vi "MenuProb.vi"(11 "Menu out":refnum<class "Menu.lvclass">) -> (2 "Value String":string, 3 "Boolean":bool)   [LabVIEW 2021, in "Menu.lvlib" / "Menu.lvclass"]
uses:
  Menu.lvclass
  Data.ctl
  Picture2D/src/Color/Color.lvclass
  Picture2D/src/Font/Font.lvclass
  Picture2D/src/Picture2D/Picture2D.lvclass
  MenuItems.ctl
  <vilib>/Utility/miscctls.llb/LVMenuShortCut.ctl
  Picture2D/src/Picture/Image.lvclass
  MenuSelection.ctl
  TD_CloseEvent.ctl
  MenuColors.ctl
  SubMenuIcon.ctl
panel:
  out "data value":T1={"MenuMap"={}, "PictRef"=refnum, "MenuSelectionEvent"=refnum, "TopMenuSpacing"=3, "MenuSpacing"=10, "CloseEvent"=refnum, "TR_ManageMenuRef"=refnum, "MenuColors"={"Text"=refnum, "HiliteText"=refnum, "Background"=refnum, "BorderColor"=refnum, "Hilite"=refnum}, "RTMPath"=path "", "RTMVIReference"=refnum, "RTMMenuReference"=refnum, "CtlRef"=refnum, "User-Specified Font"=refnum, "Desired Font"=enum."Application Font", "SubMenuIcon"=enum."LabVIEW", "SubMenuIconClosed"=refnum, "SubMenuIconOpened"=refnum}
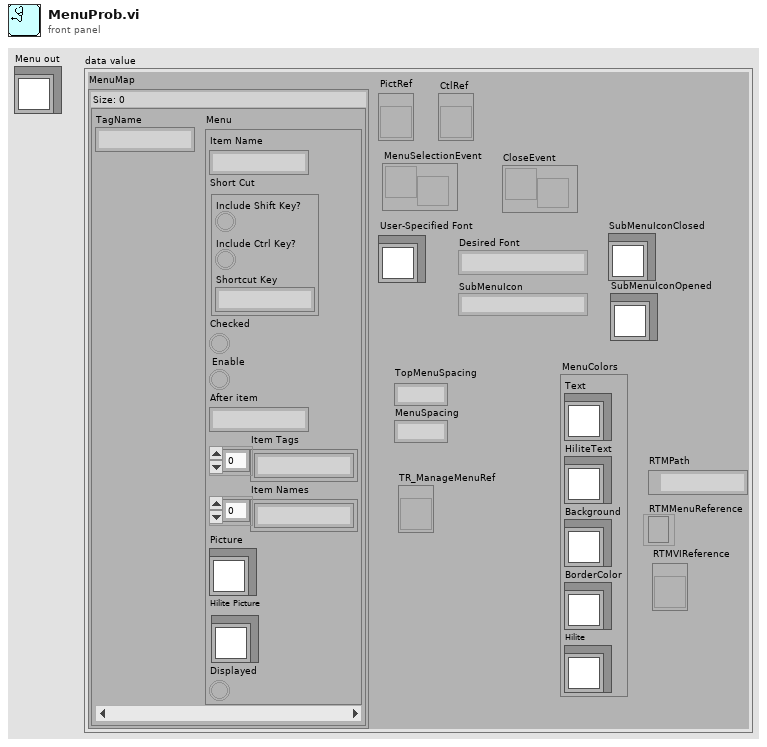
[diagram p1: front panel]
types:
  T1 = typedef "Menu.lvlib/Menu.lvclass/Data.ctl" = cluster{"MenuMap":map{string, T2}, "PictRef":refnum<vi>, "MenuSelectionEvent":refnum<user-event>, "TopMenuSpacing":i32, "MenuSpacing":i32, "CloseEvent":refnum<user-event>, "TR_ManageMenuRef":refnum<vi>, "MenuColors":T4, "RTMPath":path, "RTMVIReference":refnum<vi>, "RTMMenuReference":refnum<k9>, "CtlRef":refnum<vi>, "User-Specified Font":refnum<class "Font.lvclass">, "Desired Font":enum16{"User-specified Font", "Application Font", "System Font", "Dialog Font"}, "SubMenuIcon":T5, "SubMenuIconClosed":refnum<class "Picture2D.lvclass">, "SubMenuIconOpened":refnum<class "Picture2D.lvclass">}
  T2 = typedef "Menu.lvlib/Menu.lvclass/MenuItems.ctl" = cluster{"Item Name":string, "Short Cut":T3, "Checked":bool, "Enable":bool, "After item":string, "Item Tags":string[], "Item Names":string[], "Picture":refnum<class "Image.lvclass">, "Hilite Picture":refnum<class "Image.lvclass">, "Displayed":bool}
  T3 = typedef "LVMenuShortCut.ctl" = cluster{"Include Shift Key?":bool, "Include Ctrl Key?":bool, "Shortcut Key":string}
  T4 = typedef "Menu.lvlib/Menu.lvclass/MenuColors.ctl" = cluster{"Text":refnum<class "Color.lvclass">, "HiliteText":refnum<class "Color.lvclass">, "Background":refnum<class "Color.lvclass">, "BorderColor":refnum<class "Color.lvclass">, "Hilite":refnum<class "Color.lvclass">}
  T5 = typedef "Menu.lvlib/Menu.lvclass/SubMenuIcon.ctl" = enum16{"LabVIEW", "Windows", "Custom"}
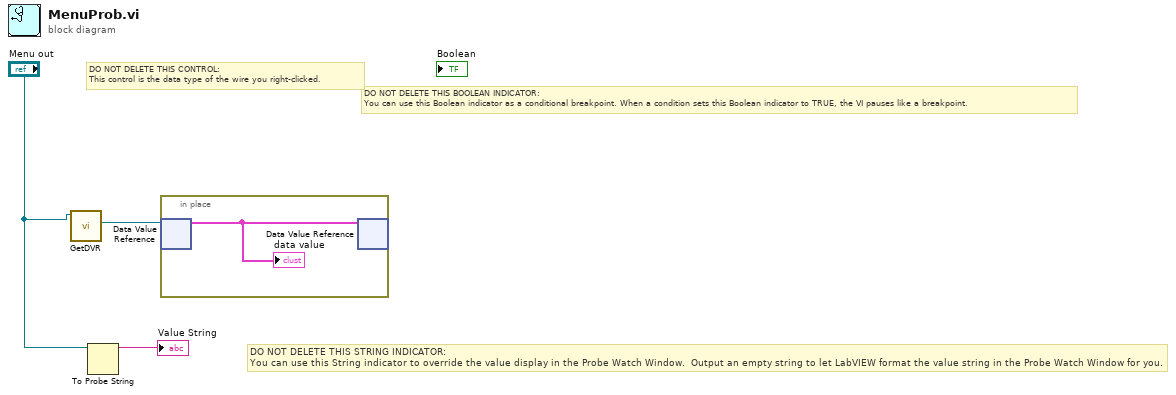
[diagram p0: block diagram]
diagram:
  # "DO NOT DELETE THIS STRING INDICATOR: \nYou can use this String indicator to override the value display in the Probe Watch Window.  Output an empty string to let LabVIEW format the value string in the Probe Watch Window for you."
  # "DO NOT DELETE THIS BOOLEAN INDICATOR: \nYou can use this Boolean indicator as a conditional breakpoint. When a condition sets this Boolean indicator to TRUE, the VI pauses like a breakpoint."
  # "DO NOT DELETE THIS CONTROL: \nThis control is the data type of the wire you right-clicked."
  n1 = call "GetDVR.vi"("Menu in"="Menu out") -> ("DVR"=w1:refnum<data-value>)  [unwired: 8 in, 2 out]
  n2 = To Probe String(7:"Menu out") -> (3:→"Value String":string)  [unwired: 2 in, 1 out]
  n3 = in-place {
    n4 = in-place-dvr #1(w1) -> (w4:T1)  [unwired: 1 out]
    "data value" <- w4
    n5 = in-place-dvr #1(w4) -> ()  [unwired: 2 out]
  }
